vi "_CheckUserLegal.vi"(8 "error in (no error)":errorcluster, 11 "Username":string) -> (0 "error out":errorcluster, 2 "Legal?":bool)   [LabVIEW 2017, in "Login-UI.lvlib"]
uses:
  Login-UI.lvlib
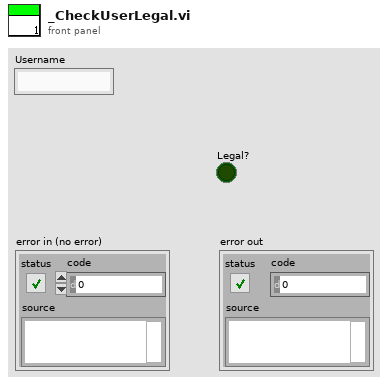
[diagram p1: front panel]
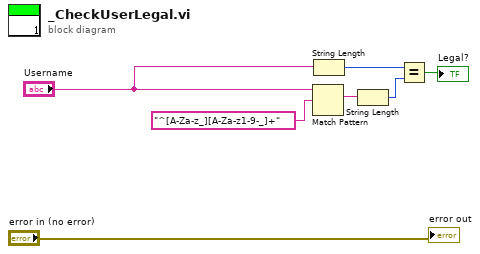
[diagram p0: block diagram]
diagram:
  n1 = Match Pattern(string="Username", regular expression="^[A-Za-z_][A-Za-z1-9-_]+") -> (match substring=w2:string)  [unwired: 1 in, 3 out]
  n2 = String Length(string="Username") -> (length=w3:i32)
  n3 = String Length(string=w2) -> (length=w1:i32)
  n4 = Equal?(x=w3, y=w1) -> (x = y?=→"Legal?":bool)
  "error out" <- "error in (no error)"
